vi "Initialize.vi"(0 "VISA resource name":refnum<visa-resource-name>, 1 "ID Query (True)":bool=TRUE, 2 "Reset (False)":bool, 3 "error in (no error)":errorcluster, 4 "Serial Link (RS232)":enum16{"RS232", "USB"}(ring)) -> (7 "VISA resource name out":refnum<visa-resource-name>, 10 "error out":errorcluster {"code" format="%.0x"})   [LabVIEW 2017, in "Newport ESP301.lvlib"]
doc: "Establishes communication with the instrument and optionally performs an instrument identification query and/or an instrument reset. It also places the instrument in a default state needed for other instrument driver operations. Therefore, call this VI before calling other instrument driver VIs for this instrument. Generally, you need to call the Initialize VI only once at the beginning of an application."
uses:
  Newport ESP301.lvlib
panel:
  # "(c) 2009 <Newport>.  ALL RIGHTS RESERVED."
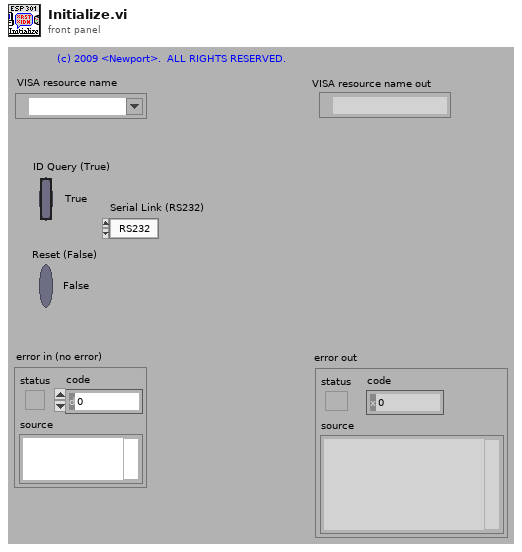
[diagram p1: front panel]
types:
  T1 = cluster{"Baud Rate":u32, "Parity":u16, "Data Bits":u16, "Stop Bits":u16, "Flow Control":u16}
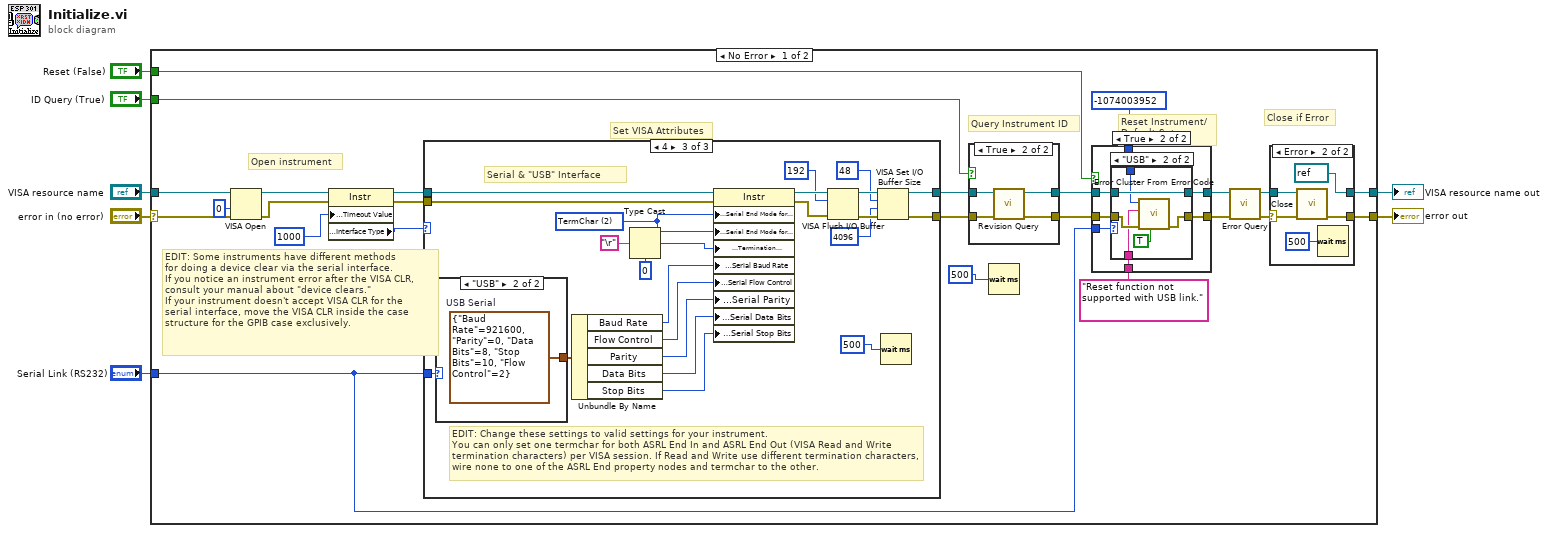
[diagram p0: block diagram]
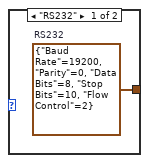
[diagram p5: hidden frame]
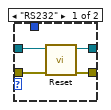
[diagram p7: hidden frame]
diagram:
  n1 = case shown="No Error" "error in (no error)" {
    selector: "error in (no error)" -> [w18 w95]
    tunnel: "ID Query (True)" -> [w30 _]
    tunnel: "Reset (False)" -> [w29 _]
    tunnel: "VISA resource name" -> [w28 w94]
    tunnel: [w14 w94] -> w4
    tunnel: [w16 w95] -> w3
    tunnel: "Serial Link (RS232)" -> [w13 _]
    frame No Error {
      # "EDIT: Some instruments have different methods\nfor doing a device clear via the serial interface.  \nIf you notice an instrument error after the VISA CLR,\nconsult your manual about \"device clears.\"  \nIf your instrument doesn't accept VISA CLR for the\nserial interface, move the VISA CLR inside the case \nstructure for the GPIB case exclusively."
      # "Set VISA Attributes"
      # "Close if Error"
      # "Query Instrument ID"
      # "Reset Instrument/\nDefault Setup"
      # "Open instrument"
      n2 = VISA Open(access mode=u32 0, error in (no error)=w18, VISA resource name=w28) -> (VISA resource name=w10:refnum<visa-resource-name>, error out=w9:errorcluster)  [unwired: 2 out]
      n3 = property class="Instr"(reference=w10, error in=w9, "General Settings:Timeout Value"=u32 1000) -> (reference out=w24:refnum<visa-resource-name>, error out=w23:errorcluster, "Interface Information:Interface Type"=w19:u16)
      n4 = case shown="4" w19 {
        tunnel: [w40 w43 w63] -> w26
        tunnel: [w41 w42 w60] -> w25
        tunnel: w24 -> [w40 w43 w65]
        tunnel: w23 -> [w41 w42 w66]
        tunnel: w13 -> [_ _ w47]
        frame Default {
          # "TCP/IP, and USB Interface"
        }
        frame 1 {
          # "GPIB Interface"
        }
        frame 4 {
          w54 = u16 2 items=["None", "LastBit", "TermChar"] ("Serial Settings:Serial End Mode for Reads")
          # "EDIT: Change these settings to valid settings for your instrument.\nYou can only set one termchar for both ASRL End In and ASRL End Out (VISA Read and Write termination characters) per VISA session. If Read and Write use different termination characters, wire none to one of the ASRL End property nodes and termchar to the other."
          # "Serial & \"USB\" Interface"
          n5 = case shown="\"USB\"" w47 {
            tunnel: [w67 w68] -> w46
            frame "RS232" {
              w67 = T1 {"Baud Rate"=19200, "Parity"=0, "Data Bits"=8, "Stop Bits"=10, "Flow Control"=2}  # RS232
            }
            frame "USB" {
              w68 = T1 {"Baud Rate"=921600, "Parity"=0, "Data Bits"=8, "Stop Bits"=10, "Flow Control"=2}  # USB Serial
            }
          }
          n6 = Unbundle By Name(w46) -> ("Baud Rate"=w52:u32, "Flow Control"=w49:u16, "Parity"=w50:u16, "Data Bits"=w51:u16, "Stop Bits"=w48:u16)
          n7 = Type Cast(type=u8 0, x="\r") -> (*(type *) &x=w53:u8)
          n8 = property class="Instr"(reference=w65, error in=w66, "Serial Settings:Serial End Mode for Reads"=w54, "Serial Settings:Serial End Mode for Writes"=w54, "Message Based Settings:Termination Character"=w53, "Serial Settings:Serial Baud Rate"=w52, "Serial Settings:Serial Flow Control"=w49, "Serial Settings:Serial Parity"=w50, "Serial Settings:Serial Data Bits"=w51, "Serial Settings:Serial Stop Bits"=w48) -> (reference out=w59:refnum<visa-resource-name>, error out=w62:errorcluster)
          n9 = VISA Flush I/O Buffer(VISA resource name=w59, mask (16)=u16 192, error in (no error)=w62) -> (VISA resource name out=w64:refnum<visa-resource-name>, error out=w61:errorcluster)
          n10 = VISA Set I/O Buffer Size(VISA resource name=w64, mask (16)=u16 48, size (4096)=u32 4096 ("size (0)"), error in (no error)=w61) -> (VISA resource name out=w63:refnum<visa-resource-name>, error out=w60:errorcluster)
          n11 = Wait (ms)(milliseconds to wait=500) -> ()  [unwired: 1 out]
        }
      }
      n12 = case shown="True" w30 {
        tunnel: [w88 w90] -> w31
        tunnel: [w89 w92] -> w32
        tunnel: w26 -> [w89 w93]
        tunnel: w25 -> [w88 w91]
        frame False {
        }
        frame True {
          n13 = call "Revision Query.vi"("error in (no error)"=w91, "VISA resource name"=w93) -> ("error out"=w90:errorcluster, "VISA resource name out"=w92:refnum<visa-resource-name>)  [unwired: 8 out]
        }
      }
      n14 = Wait (ms)(milliseconds to wait=500) -> ()  [unwired: 1 out]
      n15 = case shown="True" w29 {
        tunnel: w31 -> [w69 w74]
        tunnel: [w69 w77] -> w20
        tunnel: w32 -> [w70 w75]
        tunnel: [w70 w76] -> w21
        tunnel: w13 -> [_ w73]
        tunnel: -1074003952 ("Code") -> [_ w72]
        tunnel: "Reset function not supported with USB link." ("Source (VI Name)") -> [_ w71]
        frame False {
        }
        frame True {
          n16 = case shown="\"USB\"" w73 {
            tunnel: [w81 w84] -> w77
            tunnel: [w80 w87] -> w76
            tunnel: w75 -> [w79 w87]
            tunnel: w74 -> [w78 w85]
            tunnel: w72 -> [_ w83]
            tunnel: w71 -> [_ w82]
            frame "RS232" {
              n17 = call "Reset.vi"("error in (no error)"=w78, "VISA resource name"=w79) -> ("error out"=w81:errorcluster, "VISA resource name out"=w80:refnum<visa-resource-name>)  [unwired: 4 out]
            }
            frame "USB" {
              n18 = call <vilib>:"Error Cluster From Error Code.vi"("show call chain? (False)"=TRUE, "error in (no error)"=w85, "error message (\"\")"=w82, "error code (0)"=w83) -> ("error out"=w84:errorcluster)  [unwired: 5 out]
            }
          }
        }
      }
      n19 = call "Error Query.vi"("error in (no error)"=w20, "VISA resource name"=w21) -> ("error out"=w17:errorcluster, "VISA resource name out"=w15:refnum<visa-resource-name>)  [unwired: 4 out]
      n20 = case shown="Error" w17 {
        selector: w17 -> [w34 w37]
        tunnel: w15 -> [w33 w38]
        tunnel: [w33 refnum<visa-resource-name> refnum ("VISA resource name out")] -> w14
        tunnel: [w34 w39] -> w16
        frame No Error {
        }
        frame Error {
          n21 = call "Close.vi"("error in (no error)"=w37, "VISA resource name"=w38) -> ("error out"=w39:errorcluster)  [unwired: 9 out]
          n22 = Wait (ms)(milliseconds to wait=500) -> ()  [unwired: 1 out]
        }
      }
    }
    frame Error {
    }
  }
  "VISA resource name out" <- w4
  "error out" <- w3
